vi "小波包变换.vi"(3 "数据文件路径（输入）":string="H:\\科研项目\\仅一项目\\程序\\AI11.csv") -> (1 "特征值（输出）":dbl[][](array[numeric]))   [LabVIEW 2018]
panel:
  in  "XB_NLP2.IClass1":refnum<k7>
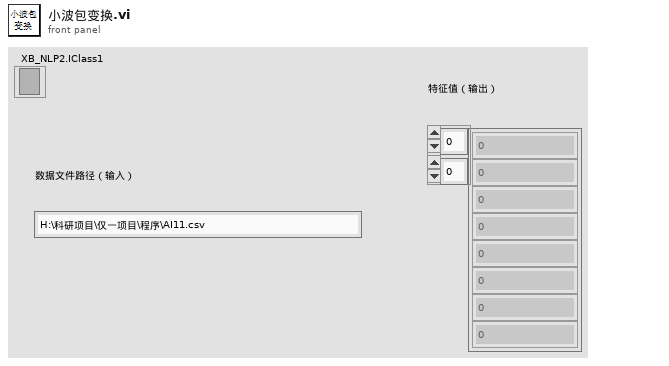
[diagram p1: front panel]
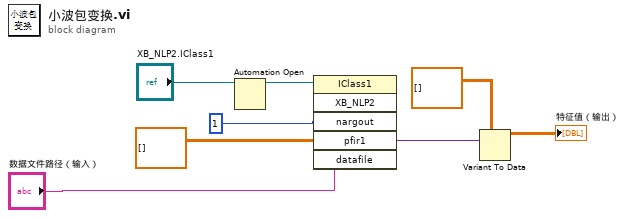
[diagram p0: block diagram]
diagram:
  n1 = Automation Open(Automation Refnum="XB_NLP2.IClass1") -> (Automation Refnum=w5:refnum<k7>)  [unwired: 3 in, 1 out]
  n2 = invoke class="IClass1" method="XB_NLP2"(reference=w5, "nargout"=1, "pfir1"=dbl[][] [] ("type"), "datafile"="数据文件路径（输入）") -> ("pfir1"=w3:variant)  [unwired: 2 in, 5 out]
  n3 = Variant To Data(type=dbl[][] [], Variant=w3) -> (data=→"特征值（输出）":dbl[][])  [unwired: 1 in, 1 out]
